vi "instance count allowed.vi"(8 "error in":errorcluster, 11 "ScaleAndLimitModule configuration in":refnum<class "ScaleAndLimitModule configuration.lvclass">) -> (0 "error out":errorcluster, 2 "instances allowed":i32, 3 "ScaleAndLimitModule configuration out":refnum<class "ScaleAndLimitModule configuration.lvclass">)   [LabVIEW 2017, in "ScaleAndLimitModule configuration.lvclass"]
uses:
  ScaleAndLimitModule configuration.lvclass
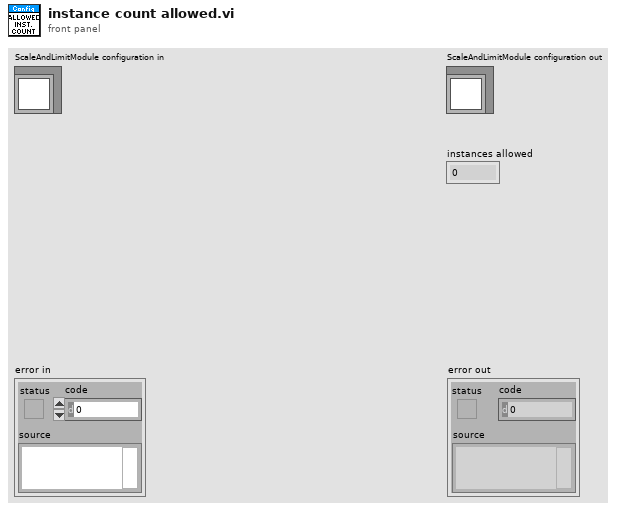
[diagram p1: front panel]
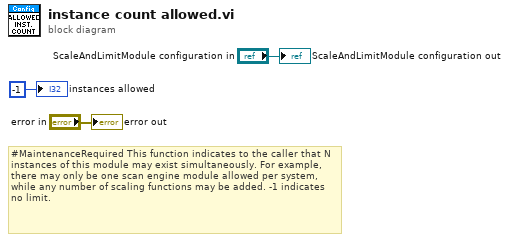
[diagram p0: block diagram]
diagram:
  # "#MaintenanceRequired This function indicates to the caller that N instances of this module may exist simultaneously. For example, there may only be one scan engine module allowed per system, while any number of scaling functions may be added. -1 indicates no limit."
  "error out" <- "error in"
  "ScaleAndLimitModule configuration out" <- "ScaleAndLimitModule configuration in"
  "instances allowed" <- -1 ("instances allowed")
